vi "Initialise Sound Effects.vi"(8 "error in (no error)":errorcluster, 11 "Main Controller Actor in":refnum<class "Main Controller Actor.lvclass">) -> (0 "error out":errorcluster, 3 "Main Controller Actor out":refnum<class "Main Controller Actor.lvclass">)   [LabVIEW 2021, in "Main Controller Actor.lvclass"]
uses:
  Main Controller Actor.lvclass
  Main Controller Actor.lvclass/Main Controller Actor.ctl
  LabSDL2/Source/Libraries/LibSDL2_Mixer Wrapper/LibSDL2_Mixer.lvlib
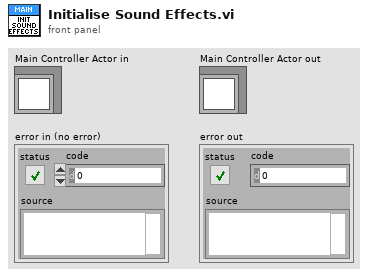
[diagram p1: front panel]
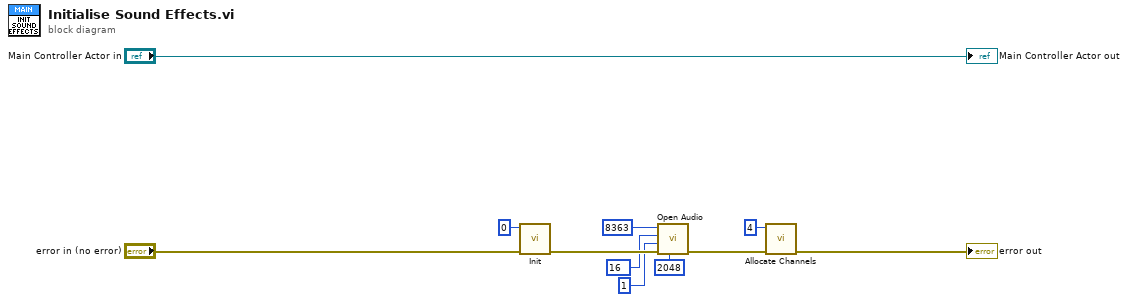
[diagram p0: block diagram]
diagram:
  n1 = call "Init.vi"("error in"="error in (no error)", "Flags"=0) -> ("error out"=w10:errorcluster)  [unwired: 8 in, 1 out]
  n2 = call "Open Audio.vi"("Chunksize"=2048, "error in"=w10, "Channels"=1, "Format"=u16 16, "Frequency"=8363) -> ("error out"=w4:errorcluster)  [unwired: 5 in, 1 out]
  n3 = call "Allocate Channels.vi"("error in"=w4, "Num Channels"=4) -> ("error out"=→"error out":errorcluster)  [unwired: 8 in, 1 out]
  "Main Controller Actor out" <- "Main Controller Actor in"
